vi "serial data communication.vi"(0 "VISA resource name":refnum<visa-resource-name>="COM1", 1 "stop bits":u16(ring)=10 items=["1.0"=10, "1.5"=15, "2.0"=20], 4 "string to write":string="*IDN?", 5 "baud rate":u32=9600, 8 "bytes to read":u32=5, 9 "data bits":u16=8 min=5 max=8 step=1, 10 "write":bool=TRUE, 11 "parity":u16(ring) items=["None", "Odd", "Even", "Mark", "Space"], 12 "flow control":u16(ring) items=["None"=0, "XON/XOFF"=1, "RTS/CTS"=2, "DTR/DSR"=4], 15 "Assert DTR?":bool=TRUE) -> (6 "read string":string)   [LabVIEW 2017]
doc: "The NI RS-485 Transceiver Control example sets the RS-485 transceiver control modes for the specified port and performs a Serial Port Read, a Serial Port Write, or a combination of these actions. If all are selected, the VI will write the data first, read data and then close the VISA session that is opened to the port. This VI will wait until the specified number of bytes is received at the port. Only the number of bytes specified will be read.\nNote: This example will work only with National Instruments RS-485 interfaces.\n\nINSTRUCTIONS:\n\n1) Select the serial resource and configuration parameters (baud rate, data bits, parity, stop bits, flow control).\n2) Set the required RS-485 transceiver mode. Set the DTR switch to the appropriate setting, depending on whether the transceiver mode is DTR controlled.\n3) Select the operations to be performed. \n4) Connect the serial port to your device. If no device is available, perform a loopback test by doing the following. Short pin 4 to pin 8 and pin 5 to pin 9 on a RS-485 cable. \n5) Run the VI to see the data read. (The \"read string\" will match the \"string to write\" if a loopback test was performed.)\n\nThis example demonstrates the transceiver control modes available when using a National Instruments RS-485 product. When connecting one or several devices via RS-485, a user may want to cut down on the amount of wiring. Alternatively, some devices offer a certain wiring configuration that you may need to match. Determine the wiring needs of the connected serial device to determine which NI RS-485 transceiver control mode to choose.\n\nNote: When you are communicating with a two-wire device, National Instruments\nrecommends that you use the two-wire Auto Control mode. Because this mode handles the transmitter/receiver enabling for a two-wire connection in your hardware, it reduces the software overhead required to perform this operation in your application program."
uses:
  <vilib>/Instr/_visa.llb/VISA Configure Serial Port (Instr).vi
panel:
  in  "CR-LF Add":bool
  out "return count":u32
  out "Write":errorcluster
  in  "Start Button":bool
  in  "string to write 2":string="*IDN?"
  out "Read":errorcluster
  in  "Button":bool
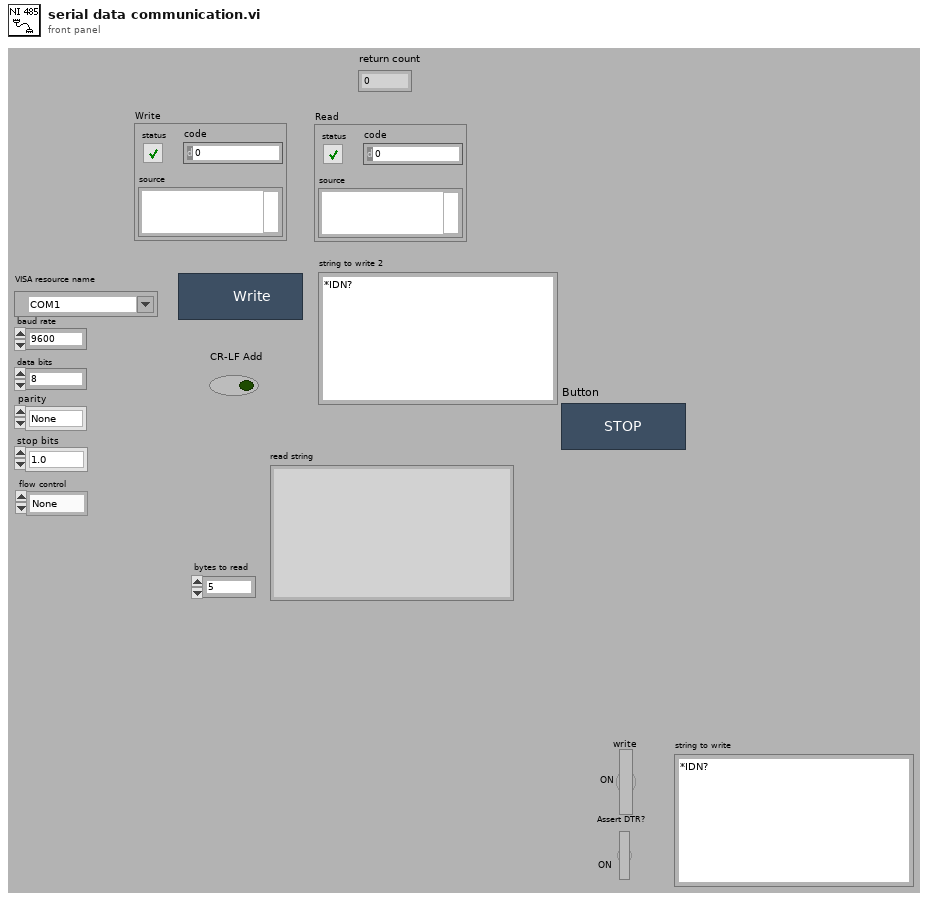
[diagram p1: front panel]
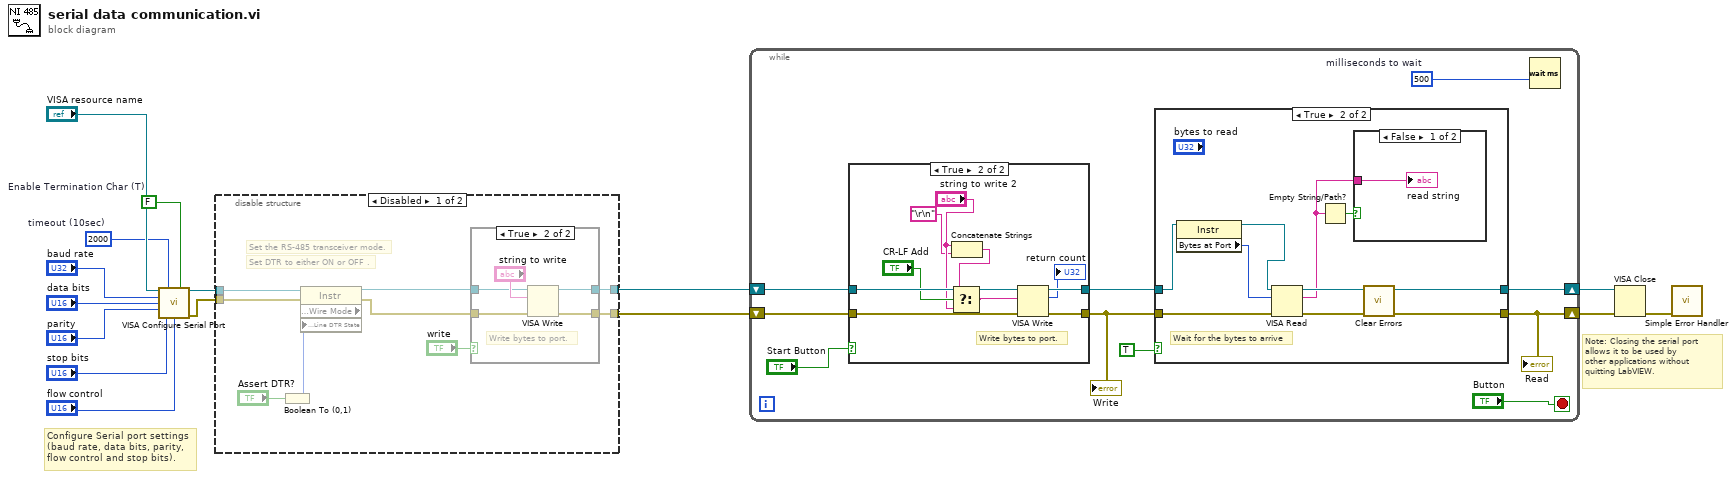
[diagram p0: block diagram]
diagram:
  w10 = FALSE  # Enable Termination Char (T)
  w3 = u32 2000  # timeout (10sec)
  # "Configure Serial port settings (baud rate, data bits, parity, flow control and stop bits)."
  # "Note: Closing the serial port\nallows it to be used by \nother applications without quitting LabVIEW."
  n1 = call-poly "VISA Configure Serial Port"("VISA resource name"="VISA resource name", "timeout (10sec)"=w3, "Enable Termination\nChar (T)"=w10, "baud rate (9600)"="baud rate", "data bits (8)"="data bits", "parity (0:none)"="parity", "stop bits (10: 1 bit)"="stop bits", "flow control (0:none)"="flow control") -> ("VISA resource name out"=w9:refnum<visa-resource-name>, "error out"=w8:errorcluster)  [unwired: 6 in]
  n2 = disable-structure shown="Disabled" {
    disable-tunnel: [w24 w34] -> w2
    disable-tunnel: w9 -> [w23 w34]
    disable-tunnel: w8 -> [w22 w33]
    disable-tunnel: [w16 w33] -> w1
    frame Disabled {
      # "Set DTR to either ON or OFF ."
      # "Set the RS-485 transceiver mode."
      n3 = Boolean To (0,1)(Boolean="Assert DTR?") -> (0, 1=w18:i16)
      n4 = property class="Instr"(reference=w23, error in=w22, "Serial Settings:Modem Line Settings:Line DTR State"=w18) -> (reference out=w19:refnum<visa-resource-name>, error out=w20:errorcluster, "Serial Settings:Wire Mode"=w17:i16)
      n5 = case shown="True" "write" {
        tunnel: [w27 w32] -> w16
        tunnel: w19 -> [w26 w30]
        tunnel: w20 -> [w27 w29]
        tunnel: [w26 w28] -> w24
        frame False {
        }
        frame True {
          # "Write bytes to port."
          n6 = VISA Write(VISA resource name=w30, write buffer="string to write", error in (no error)=w29) -> (VISA resource name out=w28:refnum<visa-resource-name>, error out=w32:errorcluster)  [unwired: 1 out]
        }
      }
    }
    frame Enabled {
    }
  }
  n7 = while {
    shift-right: [w43] -> w12
    shift-left: w2 -> [w36]
    shift-right: [w44] -> w13
    shift-left: w1 -> [w37]
    stop <- "Button" stop-if-true
    w40 = u32 500  # milliseconds to wait
    n8 = case shown="True" "Start Button" {
      tunnel: [w46 w56] -> w38
      tunnel: w36 -> [w45 w55]
      tunnel: w37 -> [w46 w54]
      tunnel: [w45 w53] -> w39
      frame False {
      }
      frame True {
        # "Write bytes to port."
        n9 = Concatenate Strings("string to write 2", "\r\n") -> (w47:string)
        n10 = Select(t=w47, s="CR-LF Add", f="string to write 2") -> (s? t:f=w51:string)
        n11 = VISA Write(VISA resource name=w55, write buffer=w51, error in (no error)=w54) -> (VISA resource name out=w53:refnum<visa-resource-name>, return count=→"return count":u32, error out=w56:errorcluster)
      }
    }
    "Write" <- w38
    n12 = case shown="True" TRUE {
      tunnel: w39 -> [w57 w60]
      tunnel: [w58 w64] -> w44
      tunnel: [w57 w66] -> w43
      tunnel: w38 -> [w58 w67]
      frame False {
      }
      frame True {
        # "Wait for the bytes to arrive"
        n13 = property class="Instr"(reference=w60) -> (reference out=w59:refnum<visa-resource-name>, "Bytes at Port"=w61:u32)  [unwired: 1 in, 1 out]
        n14 = VISA Read(VISA resource name=w59, byte count=w61, error in (no error)=w67) -> (VISA resource name out=w66:refnum<visa-resource-name>, read buffer=w63:string, error out=w65:errorcluster)  [unwired: 1 out]
        n15 = Empty String/Path?(string/path=w63) -> (empty?=w62:bool)
        n16 = case shown="False" w62 {
          tunnel: w63 -> [w68 _]
          frame False {
            "read string" <- w68
          }
          frame True {
          }
        }
        n17 = call <vilib>:"Clear Errors.vi"("error in (no error)"=w65) -> ("error out"=w64:errorcluster)  [unwired: 5 in, 1 out]
      }
    }
    "Read" <- w44
    n18 = Wait (ms)(milliseconds to wait=w40) -> ()  [unwired: 1 out]
  }
  n19 = VISA Close(VISA resource name=w12, error in (no error)=w13) -> (error out=w5:errorcluster)
  n20 = call <vilib>:"Simple Error Handler.vi"("error in (no error)"=w5) -> ()  [unwired: 4 in, 5 out]
